vi "AE - Bluetooth Rumble.vi"(8 "error in (no error)":errorcluster, 10 "Rumble?":bool=TRUE, 11 "Wiimote":u8) -> (0 "error out":errorcluster)   [LabVIEW 2011]
uses:
  AE Cores/AE - Bluetooth Enum.ctl
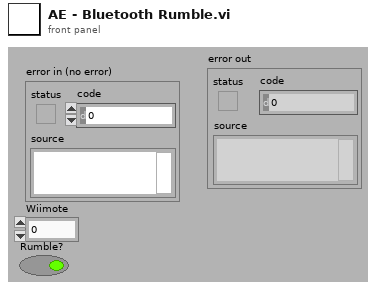
[diagram p1: front panel]
types:
  T1 = typedef "AE - Bluetooth Enum.ctl" = enum16{"Initialise", "Pair All Wiimotes", "Connect All Wiimotes", "Set Rumble", "Set LED", "Get Button + Acc Data", "Get IR Data", "Get Battery", "Get Wiimote Reference", "Reorder Wiimotes", "devReport"}
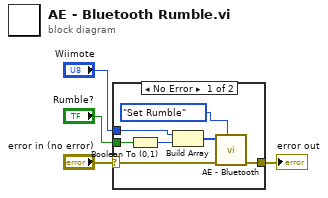
[diagram p0: block diagram]
diagram:
  n1 = case shown="No Error" "error in (no error)" {
    selector: "error in (no error)" -> [w10 w12]
    tunnel: [w9 w12] -> w3
    tunnel: "Wiimote" -> [w8 _]
    tunnel: "Rumble?" -> [w6 _]
    frame No Error {
      n2 = Boolean To (0,1)(Boolean=w6) -> (0, 1=w5:i16)
      n3 = Build Array(w8, w5) -> (w7:i16[])
      n4 = call "AE - Bluetooth.vi"("Enum"=AE_-_Bluetooth_Enum."Set Rumble", "error in (no error)"=w10, "Variant In"=w7) -> ("error out"=w9:errorcluster)  [unwired: 6 in, 2 out]
    }
    frame Error {
    }
  }
  "error out" <- w3
